vi "Variant Array to JSON Array text.vi"(5 "enable LabVIEW extensions?":bool, 6 "Pretty Print?":bool, 8 "error in (no error)":errorcluster, 10 "Array of Variants":variant[](array[variant])) -> (0 "error out":errorcluster, 3 "<JSON>":string caption="<JSON>Array")   [LabVIEW 2013, in "JSONtext.lvlib"]
uses:
  JSONtext.lvlib
  support/JSONtext support.lvlib
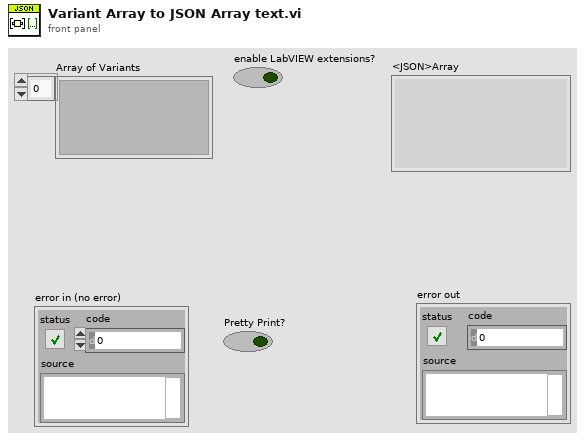
[diagram p1: front panel]
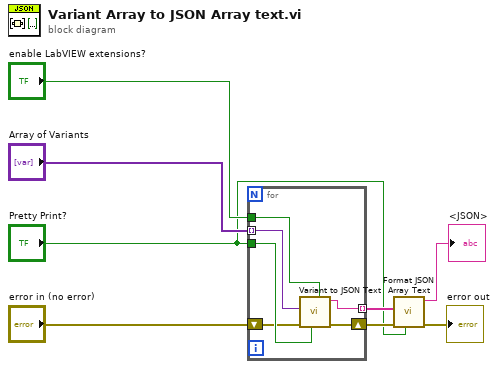
[diagram p0: block diagram]
diagram:
  n1 = for {
    tunnel: "Array of Variants" -> [w14] mode=indexing
    tunnel: "Pretty Print?" -> [w13]
    tunnel: [w9] -> w3 mode=indexing
    shift-right: [w12] -> w6
    shift-left: "error in (no error)" -> [w11]
    tunnel: "enable LabVIEW extensions?" -> [w10]
    n2 = call "Variant to JSON Text.vi"("enable LabVIEW extensions? (T)"=w10, "Pretty Print?"=w13, "error in (no error)"=w11, "Variant"=w14) -> ("error out"=w12:errorcluster, "<JSON>"=w9:string)  [unwired: 6 in]
  }
  n3 = call "Format JSON Array Text.vi"("Pretty Print?"="Pretty Print?", "error in (no error)"=w6, "Array of JSON Text"=w3) -> ("error out"=→"error out":errorcluster, "<JSON>"=→"<JSON>":string)  [unwired: 7 in]
